vi "CycleAddItem.vi"(9 "Coords":T1, 10 "动作列表框":refnum<vi>, 11 "TreeControl输入":refnum<vi>) -> (0 "添加行索引":i32, 1 "添加成功":bool, 3 "TreeControl输出":refnum<vi>)   [LabVIEW 2020, in "Curve Editor.lvlib"]
uses:
  <vilib>/Utility/miscctls.llb/LVPoint32TypeDef.ctl
  Curve Editor.lvlib
panel:
  # "将动作列表中拖曳过来的项目添加到树形列表中，并返回添加到树形后的行索引"
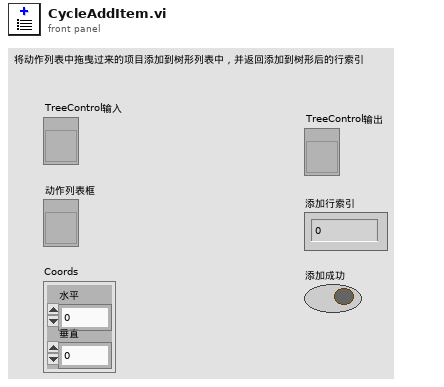
[diagram p1: front panel]
types:
  T1 = typedef "LVPoint32TypeDef.ctl" = cluster{"Horizontal":i32, "Vertical":i32}
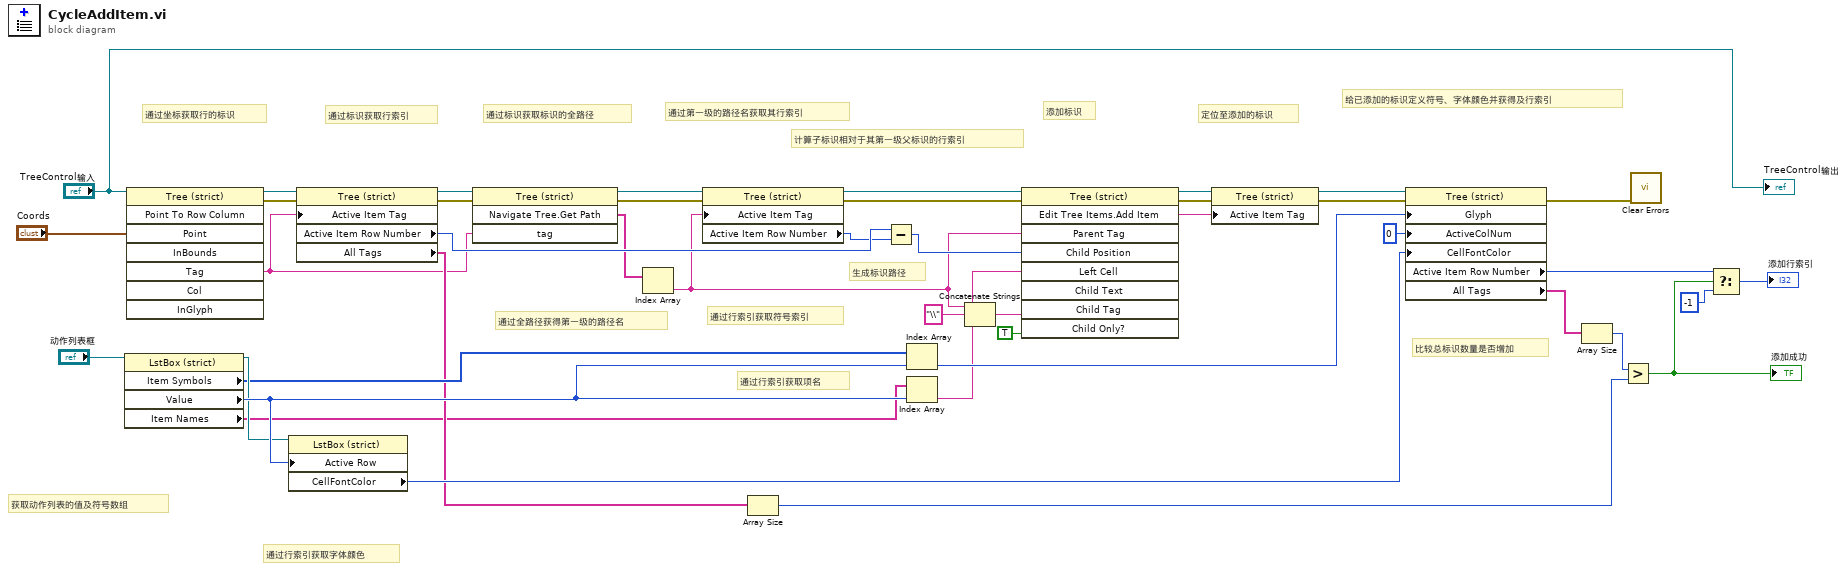
[diagram p0: block diagram]
diagram:
  # "定位至添加的标识"
  # "通过行索引获取项名"
  # "通过行索引获取符号索引"
  # "通过行索引获取字体颜色"
  # "获取动作列表的值及符号数组"
  # "比较总标识数量是否增加"
  # "给已添加的标识定义符号、字体颜色并获得及行索引"
  # "添加标识"
  # "计算子标识相对于其第一级父标识的行索引"
  # "通过第一级的路径名获取其行索引"
  # "生成标识路径"
  # "通过全路径获得第一级的路径名"
  # "通过标识获取标识的全路径"
  # "通过标识获取行索引"
  # "通过坐标获取行的标识"
  n1 = property class="LstBox (strict)"(reference="动作列表框") -> (reference out=w29:refnum<vi>, "Item Symbols"=w25:i32[], "Value"=w30:i32, "Item Names"=w14:string[])  [unwired: 1 in, 1 out]
  n2 = invoke class="Tree (strict)" method="Point To Row Column"(reference="TreeControl输入", "Point"="Coords") -> (reference out=w16:refnum<vi>, error out=w27:errorcluster, "Tag"=w17:string)  [unwired: 6 in, 5 out]
  n3 = property class="LstBox (strict)"(reference=w29, "Active Row"=w30) -> ("CellFontColor"=w31:u32)  [unwired: 1 in, 2 out]
  n4 = property class="Tree (strict)"(reference=w16, error in=w27, "Active Item Tag"=w17) -> (reference out=w23:refnum<vi>, error out=w28:errorcluster, "Active Item Row Number"=w39:i32, "All Tags"=w21:string[])
  n5 = invoke class="Tree (strict)" method="Navigate Tree.Get Path"(reference=w23, error in=w28, "tag"=w17) -> (reference out=w24:refnum<vi>, error out=w41:errorcluster, "Navigate Tree:Get Path"=w18:string[])  [unwired: 1 in, 1 out]
  n6 = Index Array(array=w18) -> (element=w37:string)  [unwired: 1 in]
  n7 = property class="Tree (strict)"(reference=w24, error in=w41, "Active Item Tag"=w37) -> (reference out=w36:refnum<vi>, error out=w42:errorcluster, "Active Item Row Number"=w38:i32)
  n8 = Array Size(array=w21) -> (size(s)=w22:i32)
  n9 = Subtract(x=w39, y=w38) -> (x-y=w40:i32)
  n10 = Index Array(array=w25, index=w30) -> (element=w13:i32)
  n11 = Index Array(array=w14, index=w30) -> (element=w10:string)
  n12 = Concatenate Strings(w37, "\\" ("字符串"), w10) -> (w12:string)
  n13 = invoke class="Tree (strict)" method="Edit Tree Items.Add Item"(reference=w36, error in=w42, "Parent Tag"=w37, "Child Position"=w40, "Left Cell"=w10, "Child Tag"=w12, "Child Only?"=TRUE ("仅作为子项？")) -> (reference out=w9:refnum<vi>, error out=w5:errorcluster, "Edit Tree Items:Add Item"=w3:string)  [unwired: 2 in, 6 out]
  n14 = property class="Tree (strict)"(reference=w9, error in=w5, "Active Item Tag"=w3) -> (reference out=w6:refnum<vi>, error out=w4:errorcluster)
  n15 = property class="Tree (strict)"(reference=w6, error in=w4, "Glyph"=w13, "ActiveColNum"=0 ("活动单元格:活动列数"), "CellFontColor"=w31) -> (error out=w26:errorcluster, "Active Item Row Number"=w33:i32, "All Tags"=w19:string[])  [unwired: 1 out]
  n16 = Array Size(array=w19) -> (size(s)=w20:i32)
  n17 = Greater?(x=w20, y=w22) -> (0:w32:bool)
  "添加成功" <- w32
  n18 = call <vilib>:"Clear Errors.vi"("error in (no error)"=w26) -> ()  [unwired: 5 in, 2 out]
  n19 = Select(t=w33, s=w32, f=-1) -> (s? t:f=→"添加行索引":i32)
  "TreeControl输出" <- "TreeControl输入"
